vi "Create Arbitrary WaveformV5.vi"(6 "Arbitrary Numeric Waveform Data":dbl[](array[numeric])=[1000.0, 2000.0, 3000.0, 4000.0, 5000.0, 6000.0, 7000.0, 8000.0], 7 "Waveform Parameters":T1={"Frequency (1000 Hz)"=1000.0, "Amplitude (2.0 Vpp)"=2.0, "DC Offset (0.00 V)"=0.0, "Phase (0.0 degrees)"=0.002} {"Phase (0.0 degrees)" min=-360.0 max=360.0 format="%#.1g"; "DC Offset (0.00 V)" min=-10.0 max=10.0; "Amplitude (2.0 Vpp)" min=0.001 max=20.0 step=1.0 format="%#.3f"; "Frequency (1000 Hz)" min=1e-06 max=160000000.0 step=1.0 format="%#.6g"}, 8 "error in (no error)":errorcluster, 9 "Select Channel (1:Channel 1)":i32(ring)=1 items=["Channel 1"=1, "Channel 2"=2], 10 "Waveform Name (\"wave1\")":string="wave1", 11 "VISA resource name":refnum<visa-resource-name>="USB0::0xF4EC::0x1101::SDG6XEBC5R0119::INSTR") -> (0 "error out":errorcluster, 3 "VISA resource name out":refnum<visa-resource-name>)   [LabVIEW 2018]
doc: "Creates and saves an arbitrary (user-defined) waveform in non-volatile memory, then selects it for output."
uses:
  <vilib>/Utility/file.llb/Read From Spreadsheet File (I64).vi
panel:
  in  "DDS/TArb 0: DDS":u16(ring) items=["DDS", "TrueArb"]
  in  "Interpolation 0: Zero-order":u16(ring) items=["Zero-Order", "Linear"]
  in  "WFM Length":i32=15
  in  "WFM (Column) Number":i32
  in  "WFM Path":path
  in  "WFM Source":u16(ring) items=["Single file", "Split files", "Array"]
  # "Wavedata accepeted: 4B~40MB"
  # "IF WFM is set to 0 (or no file selected) and single file is used, \nneeds to be power reset, as crashed!! \n(not needed when using inbuilt array)"
  # "ON run will:\nupload file\nchange to arb wavefunction\nUse uploaded waveform"
  # "For TrueArb Interpolation, TARB needed"
  # "Max value for array: 32767"
  # "Array needs to be intgers\nMax 20M points"
  # "Negative numbers are using little-endian"
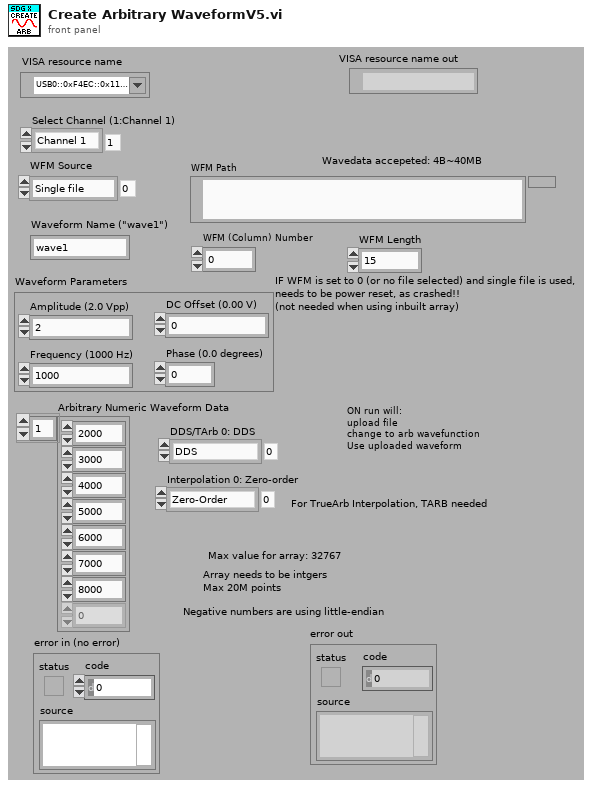
[diagram p1: front panel]
types:
  T1 = cluster{"Frequency (1000 Hz)":dbl, "Amplitude (2.0 Vpp)":dbl, "DC Offset (0.00 V)":dbl, "Phase (0.0 degrees)":dbl}
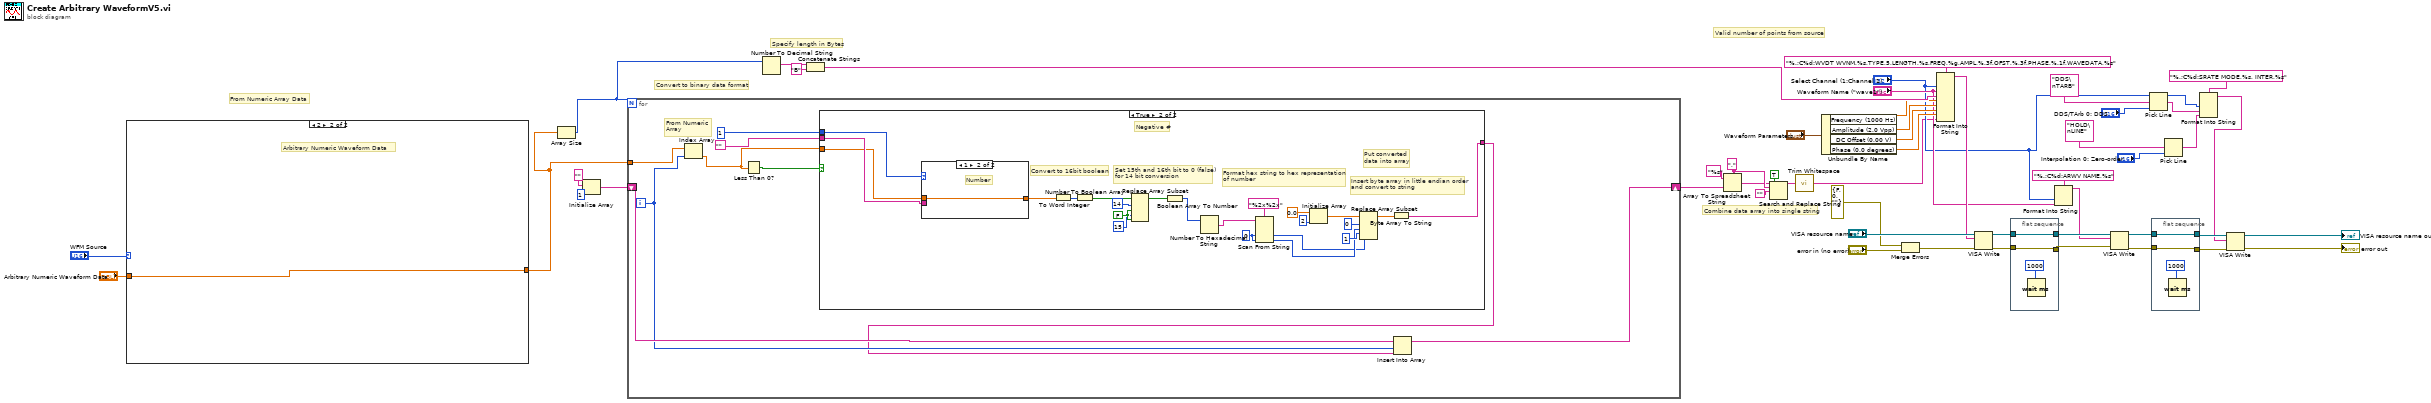
[diagram p0: block diagram]
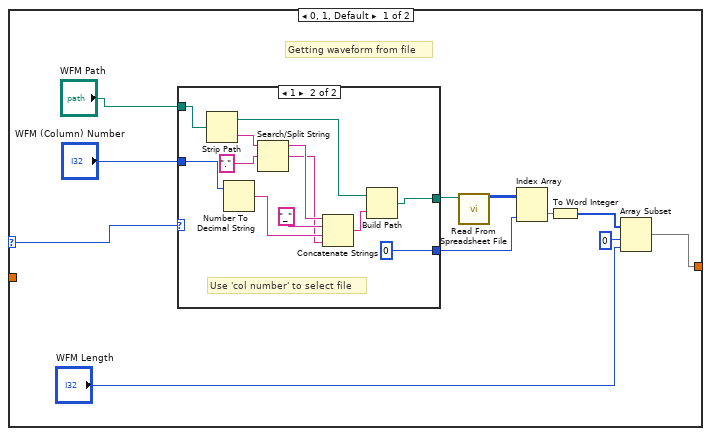
[diagram p2: hidden frame]
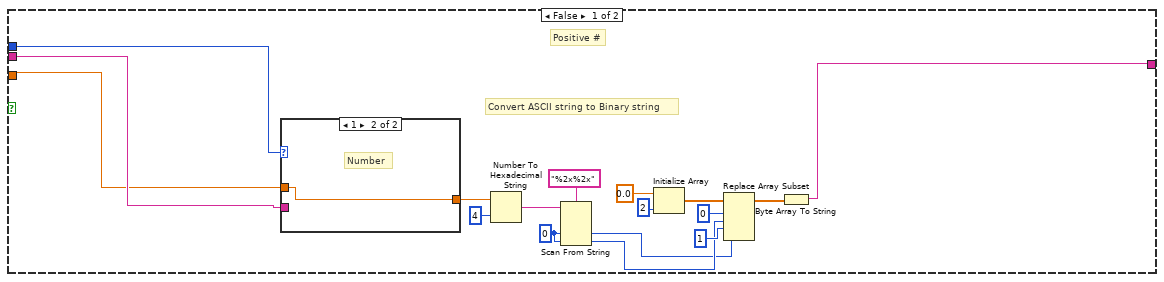
[diagram p4: hidden frame]
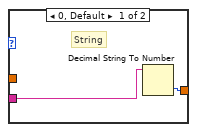
[diagram p5: hidden frame]
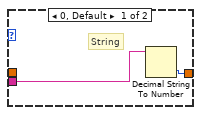
[diagram p6: hidden frame]
diagram:
  w39 = ","
  # "From Numeric Array Data"
  # "Specify length in Bytes"
  # "Combine data array into single string"
  # "Valid number of points from source"
  # "Convert to binary data format"
  n1 = case shown="2" "WFM Source" {
    selector: "WFM Source" -> [w57 _]
    tunnel: [w52 w77] -> w19
    tunnel: "Arbitrary Numeric Waveform Data" -> [_ w77]
    frame 0, 1, Default {
      # "Getting waveform from file"
      n2 = case shown="1" w57 {
        tunnel: "WFM Path" -> [w64 w76]
        tunnel: "WFM (Column) Number" -> [w63 w73]
        tunnel: [w64 w66] -> w55
        tunnel: [w63 0 ("x")] -> w54
        frame 0, Default {
          # "File contains multiple wfms"
        }
        frame 1 {
          # "Use 'col number' to select file"
          n3 = Strip Path(path=w76) -> (stripped path=w68:path, name=w74:string)
          n4 = Number To Decimal String(number=w73) -> (decimal integer string=w70:string)  [unwired: 1 in]
          n5 = Search/Split String(string=w74, search string/char (-)=".") -> (substring before match=w72:string, match + rest of string=w69:string)  [unwired: 1 in, 1 out]
          n6 = Concatenate Strings(w72, "_", w70, w69) -> (w67:string)
          n7 = Build Path(base path=w68, name or relative path=w67) -> (appended path=w66:path)
        }
      }
      n8 = call-poly <vilib>:"Read From Spreadsheet File.vi"("file path (dialog if empty)"=w55) -> ("all rows"=w56:i64[][])  [unwired: 6 in, 4 out]
      n9 = Index Array(array=w56, index (col)=w54) -> (element=w53:i64[])  [unwired: 1 in]
      n10 = To Word Integer(number=w53) -> (16bit integer=w62:i16[])
      n11 = Array Subset(array=w62, index=0 ("x"), length="WFM Length") -> (w52:i16[])
    }
    frame 2 {
      # "Arbitrary Numeric Waveform Data"
    }
  }
  n12 = Array Size(array=w19) -> (size(s)=w20:i32)
  n13 = Initialize Array("", 1) -> (w43:string[])
  n14 = for {
    N: w20 -> [_]
    tunnel: w19 -> [w82]
    shift-right: [w78] -> w26
    shift-left: w43 -> [w81]
    i -> [w80]
    # "From Numeric\nArray"
    # "Put converted\ndata into array"
    n15 = Index Array(array=w82, index=w80) -> (element=w85:dbl)
    n16 = Less Than 0?(x=w85) -> (x < 0?=w86:bool)
    n17 = case shown="True" w86 {
      tunnel: w85 -> [w87 w108]
      tunnel: [w88 w109] -> w79
      tunnel: "" -> [w89 w110]
      tunnel: u16 1 -> [w90 w111]
      frame False {
        w99 = 0 ("default value 1")
        # "Convert ASCII string to Binary string"
        # "Positive #"
        n18 = case shown="1" w90 {
          tunnel: [w105 w106] -> w100
          tunnel: w89 -> [w104 _]
          tunnel: w87 -> [_ w106]
          frame 0, Default {
            # "String"
            n19 = Decimal String To Number(string=w104) -> (number=w105:i32)  [unwired: 2 in, 1 out]
          }
          frame 1 {
            # "Number"
          }
        }
        n20 = Number To Hexadecimal String(1:i16 4 ("width (-)"), 2:w100) -> (0:w102:string)
        n21 = Scan From String(format string="%2x%2x", input string=w102, default 1=w99, default 2=w99) -> (output 1=w91:i32, output 2=w92:i32)  [unwired: 2 in, 3 out]
        n22 = Initialize Array(0.0 ("element"), 2) -> (w97:dbl[])
        n23 = Replace Array Subset(array=w97, new element #1=w92, index #1=0, new element #2=w91, index #2=1) -> (w94:dbl[])
        n24 = Byte Array To String(unsigned byte array=w94) -> (string=w88:string)
      }
      frame True {
        w122 = 0 ("default value 1")
        w128 = FALSE
        # "Insert byte array in little endian order\nand convert to string"
        # "Format hex string to hex representation\nof number"
        # "Set 15th and 16th bit to 0 (false)\nfor 14 bit conversion"
        # "Convert to 16bit boolean"
        # "Negative #"
        n25 = case shown="1" w111 {
          tunnel: [w131 w132] -> w112
          tunnel: w110 -> [w130 _]
          tunnel: w108 -> [_ w132]
          frame 0, Default {
            # "String"
            n26 = Decimal String To Number(string=w130) -> (number=w131:i32)  [unwired: 2 in, 1 out]
          }
          frame 1 {
            # "Number"
          }
        }
        n27 = To Word Integer(number=w112) -> (16bit integer=w129:i16)
        n28 = Number To Boolean Array(number=w129) -> (Boolean array=w125:bool[])
        n29 = Replace Array Subset(array=w125, new element #1=w128, index #1=14, new element #2=w128, index #2=15) -> (w107:bool[])
        n30 = Boolean Array To Number(Boolean array=w107) -> (number=w124:u32)
        n31 = Number To Hexadecimal String(2:w124) -> (0:w113:string)  [unwired: 1 in]
        n32 = Scan From String(format string="%2x%2x", input string=w113, default 1=w122, default 2=w122) -> (output 1=w114:i32, output 2=w115:i32)  [unwired: 2 in, 3 out]
        n33 = Initialize Array(0.0 ("element"), 2) -> (w120:dbl[])
        n34 = Replace Array Subset(array=w120, new element #1=w115, index #1=0, new element #2=w114, index #2=1) -> (w117:dbl[])
        n35 = Byte Array To String(unsigned byte array=w117) -> (string=w109:string)
      }
    }
    n36 = Insert Into Array(array=w81, index=w80, new element=w79) -> (w78:string[])
  }
  n37 = Number To Decimal String(number=w20) -> (decimal integer string=w34:string)  [unwired: 1 in]
  n38 = Concatenate Strings(w34, "B" ("string")) -> (w32:string)
  n39 = Array To Spreadsheet String(delimiter (Tab)=w39, array=w26, 3:"%s") -> (spreadsheet string=w36:string)
  n40 = Search and Replace String(replace all?=TRUE, input string=w36, search string=w39, replace string="") -> (result string=w37:string)  [unwired: 4 in, 3 out]
  n41 = call <vilib>:"Trim Whitespace.vi"("string"=w37) -> ("trimmed string"=w1:string)  [unwired: 1 in]
  n42 = Unbundle By Name("Waveform Parameters") -> ("Frequency (1000 Hz)"=w31:dbl, "Amplitude (2.0 Vpp)"=w30:dbl, "DC Offset (0.00 V)"=w29:dbl, "Phase (0.0 degrees)"=w28:dbl)
  n43 = Merge Errors(errorcluster {"status"=FALSE, "code"=0, "source"=""} ("error constant"), "error in (no error)") -> (w47:errorcluster)
  n44 = Format Into String(format string="%.;C%d:WVDT WVNM,%s,TYPE,5,LENGTH,%s,FREQ,%g,AMPL,%.3f,OFST,%.3f,PHASE,%.1f,WAVEDATA,%s", "Select Channel (1:Channel 1)", "Waveform Name (\"wave1\")", w32, w31, w30, w29, w28, w1) -> (resulting string=w50:string)  [unwired: 2 in, 1 out]
  n45 = VISA Write(VISA resource name="VISA resource name", write buffer=w50, error in (no error)=w47) -> (VISA resource name out=w25:refnum<visa-resource-name>, error out=w24:errorcluster)  [unwired: 1 out]
  n46 = flat-sequence {
    tunnel: w25 -> [w134]
    tunnel: w24 -> [w133]
    tunnel: [w134] -> w23
    tunnel: [w133] -> w22
    frame #0 {
      n47 = Wait (ms)(milliseconds to wait=1000 ("x")) -> ()  [unwired: 1 out]
    }
  }
  n48 = Format Into String(format string="%.;C%d:ARWV NAME,%s", "Select Channel (1:Channel 1)", "Waveform Name (\"wave1\")") -> (resulting string=w17:string)  [unwired: 2 in, 1 out]
  n49 = VISA Write(VISA resource name=w23, write buffer=w17, error in (no error)=w22) -> (VISA resource name out=w16:refnum<visa-resource-name>, error out=w15:errorcluster)  [unwired: 1 out]
  n50 = Pick Line(multi-line string="DDS\nTARB", line index="DDS/TArb 0: DDS") -> (output string=w2:string)  [unwired: 1 in]
  n51 = flat-sequence {
    tunnel: w16 -> [w137]
    tunnel: w15 -> [w136]
    tunnel: [w137] -> w13
    tunnel: [w136] -> w12
    frame #0 {
      n52 = Wait (ms)(milliseconds to wait=1000 ("x")) -> ()  [unwired: 1 out]
    }
  }
  n53 = Pick Line(multi-line string="HOLD\nLINE", line index="Interpolation 0: Zero-order") -> (output string=w5:string)  [unwired: 1 in]
  n54 = Format Into String(format string="%.;C%d:SRATE MODE,%s, INTER,%s", "Select Channel (1:Channel 1)", w2, w5) -> (resulting string=w6:string)  [unwired: 2 in, 1 out]
  n55 = VISA Write(VISA resource name=w13, write buffer=w6, error in (no error)=w12) -> (VISA resource name out=→"VISA resource name out":refnum<visa-resource-name>, error out=→"error out":errorcluster)  [unwired: 1 out]
